vi "Util_ConvertStringToArrayOfStrings.vi"(1 "String":string) -> (0 "Array<string>":string[](array[string]))   [LabVIEW 2020]
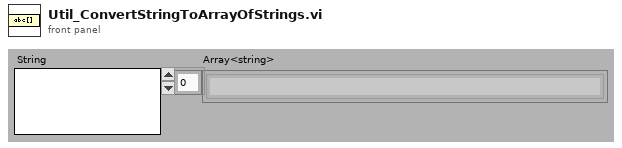
[diagram p1: front panel]
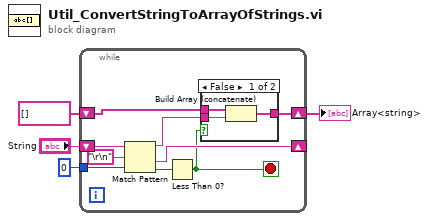
[diagram p0: block diagram]
diagram:
  n1 = while {
    shift-right: [w11] -> _
    shift-left: "String" -> [w13]
    tunnel: 0 -> [w9]
    shift-right: [w7] -> w2
    shift-left: string[] [] -> [w6]
    stop <- w5 stop-if-true
    n2 = Match Pattern(string=w13, regular expression="\r\n", offset (0)=w9) -> (before substring=w8:string, after substring=w11:string, offset past match=w10:i32)  [unwired: 1 out]
    n3 = Less Than 0?(x=w10) -> (x < 0?=w5:bool)
    n4 = case shown="False" w5 {
      tunnel: w8 -> [w16 _]
      tunnel: [w15 w17] -> w7
      tunnel: w6 -> [w14 w17]
      frame False {
        n5 = Build Array (concatenate)(w14, w16) -> (w15:string[])
      }
      frame True {
      }
    }
  }
  "Array<string>" <- w2
